vi "Set Error Queue.vi"(10 "Error Queue":T1, 11 "Interface in":refnum<class "Interface.lvclass">) -> (3 "Interface out":refnum<class "Interface.lvclass">)   [LabVIEW 2017, in "DSF Core.lvlib" / "Interface.lvclass"]
uses:
  Interface.lvclass
  Error Queue Ref.ctl
  Interface.lvclass/Interface.ctl
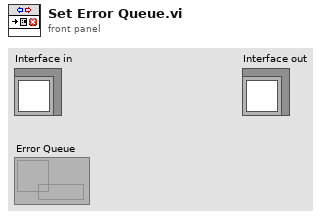
[diagram p1: front panel]
types:
  T1 = typedef "DSF Core.lvlib/Interface.lvclass/Error Queue Ref.ctl" = refnum<queue>
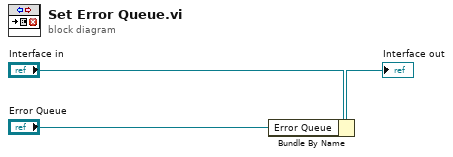
[diagram p0: block diagram]
diagram:
  n1 = Bundle By Name(cluster="Interface in", "Error Queue"="Error Queue") -> (→"Interface out":refnum<class "Interface.lvclass">)
